vi "FT_Write_EEPROM_User_Area.vi"(1 "User Area Data In":u8[](array[numeric]) format="%x", 2 "Handle":u32) -> (0 "FT_Status":u32(ring) items=["FT_OK", "FT_INVALID_HANDLE", "FT_DEVICE_NOT_FOUND", "FT_DEVICE_NOT_OPENED", "FT_IO_ERROR", "FT_INSUFFICIENT_RESOURCES", "FT_INVALID_PARAMETER", "FT_INVALID_BAUD_RATE", "FT_DEVICE_NOT_OPENED_FOR_ERASE", "FT_DEVICE_NOT_OPENED_FOR_WRITE", "FT_FAILED_TO_WRITE_DEVICE", "FT_EEPROM_READ_FAILED", "FT_EEPROM_WRITE_FAILED", "FT_EEPROM_ERASE_FAILED", "FT_EEPROM_NOT_PRESENT", "FT_EEPROM_NOT_PROGRAMMED", "FT_INVALID_ARGS", "FT_NOT_SUPPORTED", "FT_OTHER_ERROR"])   [LabVIEW 2019, in "D2XX_Functions.lvlib"]
uses:
  <userlib>/LevyLab/Relay Box/D2XX_Functions/D2XX_Functions.lvlib
  <userlib>/LevyLab/Relay Box/D2XX_Functions/i386/ftd2xx.dll
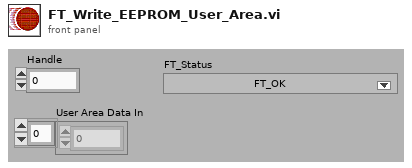
[diagram p1: front panel]
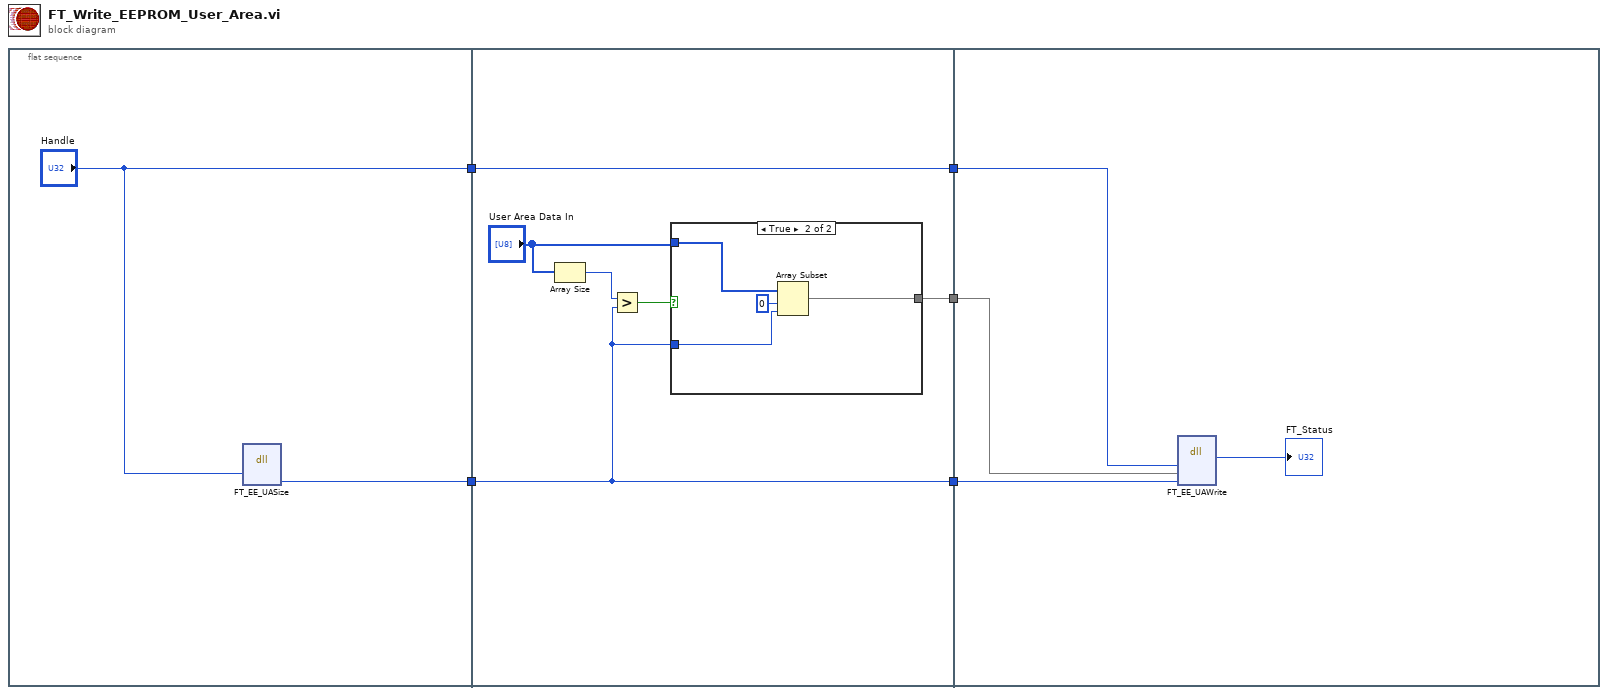
[diagram p0: block diagram]
diagram:
  n1 = flat-sequence {
    tunnel: ["Handle"] -> w5
    tunnel: [w6] -> w3
    tunnel: w5 -> [w13]
    tunnel: [w13] -> w4
    tunnel: w3 -> [w8]
    tunnel: [w8] -> w2
    tunnel: [w9] -> w1
    tunnel: w4 -> [w19]
    tunnel: w2 -> [w21]
    tunnel: w1 -> [w20]
    frame #0 {
      n2 = dll-call lib="C:/Program Files (x86)/National Instruments/LabVIEW 2019/user.lib/LevyLab/Relay Box/D2XX_Functions/i386/FTD2XX.dll" fn="FT_EE_UASize"("Handle"="Handle") -> ("UASize"=w6:u32)  [unwired: 6 in, 2 out]
    }
    frame #1 {
      n3 = Array Size(array="User Area Data In") -> (size(s)=w11:i32)
      n4 = Greater?(x=w11, y=w8) -> (0:w12:bool)
      n5 = case shown="True" w12 {
        tunnel: "User Area Data In" -> [w14 w18]
        tunnel: w8 -> [_ w15]
        tunnel: [w14 w16] -> w9
        frame False {
        }
        frame True {
          n6 = Array Subset(array=w18, index=u16 0, length=w15) -> (w16:u8[])
        }
      }
    }
    frame #2 {
      n7 = dll-call lib="C:/Program Files (x86)/National Instruments/LabVIEW 2019/user.lib/LevyLab/Relay Box/D2XX_Functions/i386/FTD2XX.dll" fn="FT_EE_UAWrite"("Handle"=w19, "Buffer"=w20, "DataLength"=w21) -> ("FT_Status"=→"FT_Status":u32)  [unwired: 6 in, 2 out]
    }
  }
